vi "Samsung Data Wrapper.vi"(7 "# Racks":i32=1, 8 "Error In":errorcluster, 10 "Samsung Data In":u16[](array[numeric]) format="%.0x") -> (0 "Error Out":errorcluster, 1 "Energy Storage System Data Out":T4={"Voltage"=0.0, "Current"=0.0, "SOC Avg"=0.0, "Faults"=0, "Alarms"=0, "# Strings"=0, "Max Temp"=0, "Min Temp"=0, "Max Cell Voltage"=0.0, "Min Cell Voltage"=0.0, "Energy Capacity"=0.0, "Energy Remaining"=0.0, "SOC Min"=0.0, "SOC Max"=0.0, "ES Fault"=FALSE, "String Select"=enum."3 Strings", "ES Com Fault"=FALSE, "SOH Avg"=0.0}, 2 "Energy Storage String Data Out":T1, 3 "Current Limit Parameters Out":T3 {"Min Cell Voltage Actual Value" format="%#.2f"; "Max Cell Voltage Actual Value" format="%#.2f"}, 5 "Contactor CMD":bool[](array[boolean]))   [LabVIEW 2014]
uses:
  Controls/ES System Data.ctl
  Controls/StringSelector.ctl
  Controls/Current Limit Parameters.ctl
  Controls/ES String Array.ctl
  Controls/ES String Data.ctl
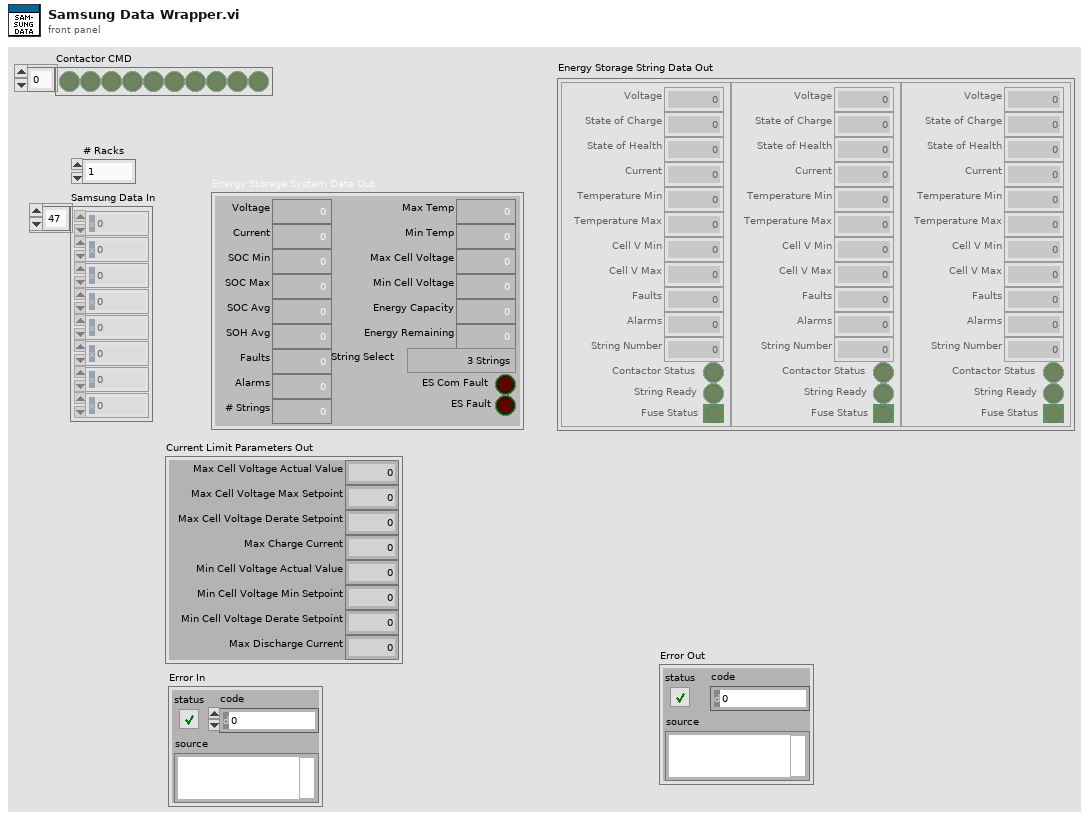
[diagram p1: front panel]
types:
  T1 = typedef "ES String Array.ctl" = T2[]
  T2 = typedef "ES String Data.ctl" = cluster{"Voltage":sgl, "State of Charge":sgl, "Current":sgl, "Temperature Min":i16, "Temperature Max":i16, "Faults":u16, "Alarms":u16, "String Number":u16, "Contactor Status":bool, "String Ready":bool, "Fuse Status":bool, "Cell V Max":dbl, "Cell V Min":dbl, "State of Health":sgl}
  T3 = typedef "Current Limit Parameters.ctl" = cluster{"Max Cell Voltage Max Setpoint":dbl, "Max Cell Voltage Actual Value":dbl, "Max Cell Voltage Derate Setpoint":dbl, "Max Charge Current":dbl, "Min Cell Voltage Min Setpoint":dbl, "Min Cell Voltage Actual Value":dbl, "Min Cell Voltage Derate Setpoint":dbl, "Max Discharge Current":dbl}
  T4 = typedef "ES System Data.ctl" = cluster{"Voltage":sgl, "Current":sgl, "SOC Avg":sgl, "Faults":u16, "Alarms":u16, "# Strings":u16, "Max Temp":i16, "Min Temp":i16, "Max Cell Voltage":sgl, "Min Cell Voltage":sgl, "Energy Capacity":sgl, "Energy Remaining":sgl, "SOC Min":sgl, "SOC Max":sgl, "ES Fault":bool, "String Select":T5, "ES Com Fault":bool, "SOH Avg":sgl}
  T5 = typedef "StringSelector.ctl" = enum16{"1 String (1)", "1 String (2)", "1 String (3)", "2 Strings (1 2)", "2 Strings (2 3)", "2 Strings (1 3)", "3 Strings"}
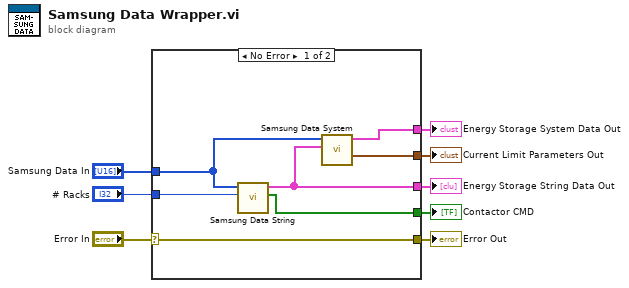
[diagram p0: block diagram]
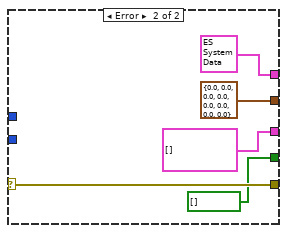
[diagram p2: hidden frame]
diagram:
  n1 = case shown="No Error" "Error In" {
    selector: "Error In" -> [w15 w20]
    tunnel: "Samsung Data In" -> [w10 _]
    tunnel: [w12 T4 {"Voltage"=0.0, "Current"=0.0, "SOC Avg"=0.0, "Faults"=0, "Alarms"=0, "# Strings"=0, "Max Temp"=0, "Min Temp"=0, "Max Cell Voltage"=0.0, "Min Cell Voltage"=0.0, "Energy Capacity"=0.0, "Energy Remaining"=0.0, "SOC Min"=0.0, "SOC Max"=0.0, "ES Fault"=FALSE, "String Select"=enum."1 String (1)", "ES Com Fault"=TRUE, "SOH Avg"=0.0} ("Energy Storage System Data")] -> w6
    tunnel: [w13 T2[] []] -> w3
    tunnel: [w11 T3 {"Max Cell Voltage Max Setpoint"=0.0, "Max Cell Voltage Actual Value"=0.0, "Max Cell Voltage Derate Setpoint"=0.0, "Max Charge Current"=0.0, "Min Cell Voltage Min Setpoint"=0.0, "Min Cell Voltage Actual Value"=0.0, "Min Cell Voltage Derate Setpoint"=0.0, "Max Discharge Current"=0.0} ("Current Limit Parameters")] -> w5
    tunnel: [w15 w20] -> w4
    tunnel: "# Racks" -> [w14 _]
    tunnel: [w9 bool[] [] ("Contactor CMD")] -> w1
    frame No Error {
      n2 = call "Samsung Data String.vi"("# Racks"=w14, "Samsung Data In"=w10) -> ("Contactor CMD"=w9:bool[], "Samsung String Data Array"=w13:T2[])  [unwired: 8 in]
      n3 = call "Samsung Data System.vi"("Samsung String Data In"=w13, "Samsung Data In"=w10) -> ("Current Limit Parameters"=w11:T3, "Samsung System Data Out"=w12:T4)  [unwired: 8 in]
    }
    frame Error {
    }
  }
  "Energy Storage System Data Out" <- w6
  "Current Limit Parameters Out" <- w5
  "Error Out" <- w4
  "Energy Storage String Data Out" <- w3
  "Contactor CMD" <- w1
